vi "tabs to returns.vi"(1 "string containing tabs":string) -> (0 "string with tabs replaced with returns":string)   [LabVIEW 2015]
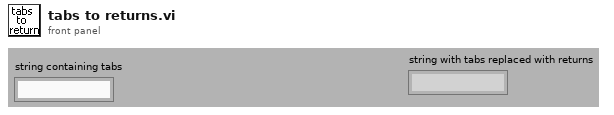
[diagram p1: front panel]
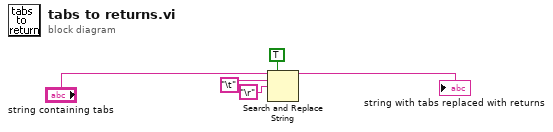
[diagram p0: block diagram]
diagram:
  n1 = Search and Replace String(replace all?=TRUE, input string="string containing tabs", search string="\t", replace string="\r") -> (result string=→"string with tabs replaced with returns":string)  [unwired: 4 in, 3 out]
